vi "Msg Receive.vi"(11 "Self Actor in":refnum<class "Self Actor.lvclass">) -> (0 "error out":errorcluster, 1 "Destroyed Self?":bool, 3 "Self Actor out":refnum<class "Self Actor.lvclass">)   [LabVIEW 2021, in "LVCAM.lvlib" / "Self Actor.lvclass"]
uses:
  Self Actor.lvclass
  Msg Q/Msg Q.lvclass
  Msgs/LVCAM Nest Destroyed/LVCAM Nest Destroyed Msg/LVCAM Nest Destroyed Msg.lvclass
  Msg/Msg.lvclass
  C:/PPLs/LabVIEW-Composed-Actor-Model-LVCAM/LabVIEW-Composed-Actor-Model-LVCAM/AAM/Msgs/LVCAM Nest Destroyed/LVCAM Nest Destroyed Msg/LVCAM Nest Destroyed Msg.lvclass
  C:/PPLs/LabVIEW-Composed-Actor-Model-LVCAM/LabVIEW-Composed-Actor-Model-LVCAM/AAM/Msgs/LVCAM Nest Destroyed/LVCAM Nest Destroyed/LVCAM Nest Destroyed.lvclass
  C:/PPLs/LabVIEW-Composed-Actor-Model-LVCAM/LabVIEW-Composed-Actor-Model-LVCAM/AAM/LVCAM/Msg/Msg.lvclass
  C:/PPLs/LabVIEW-Composed-Actor-Model-LVCAM/LabVIEW-Composed-Actor-Model-LVCAM/AAM/LVCAM/LVCAM/LVCAM.lvclass
  C:/PPLs/LabVIEW-Composed-Actor-Model-LVCAM/LabVIEW-Composed-Actor-Model-LVCAM/AAM/Msgs/LVCAM Create Nest/LVCAM Create Nest/LVCAM Create Nest.lvclass
  C:/PPLs/LabVIEW-Composed-Actor-Model-LVCAM/LabVIEW-Composed-Actor-Model-LVCAM/AAM/Msgs/LVCAM Destroy Self/LVCAM Destroy Self/LVCAM Destroy Self.lvclass
  C:/PPLs/LabVIEW-Composed-Actor-Model-LVCAM/LabVIEW-Composed-Actor-Model-LVCAM/AAM/LVCAM/Msg Receive/Msg Receive.lvclass
  C:/PPLs/LabVIEW-Composed-Actor-Model-LVCAM/LabVIEW-Composed-Actor-Model-LVCAM/AAM/LVCAM/Msg Remain/Msg Remain.lvclass
  C:/PPLs/LabVIEW-Composed-Actor-Model-LVCAM/LabVIEW-Composed-Actor-Model-LVCAM/AAM/LVCAM/Propagate Error/Propagate Error.lvclass
  C:/PPLs/LabVIEW-Composed-Actor-Model-LVCAM/LabVIEW-Composed-Actor-Model-LVCAM/AAM/LVCAM/Self Actor Decorator/Self Actor Decorator.lvclass
  C:/PPLs/LabVIEW-Composed-Actor-Model-LVCAM/LabVIEW-Composed-Actor-Model-LVCAM/AAM/LVCAM/Read Self Actor/Read Self Actor.lvclass
  C:/PPLs/LabVIEW-Composed-Actor-Model-LVCAM/LabVIEW-Composed-Actor-Model-LVCAM/AAM/LVCAM/Self Actor/Self Actor.lvclass
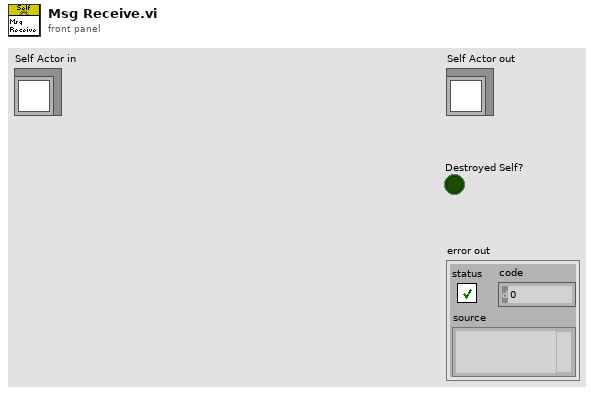
[diagram p1: front panel]
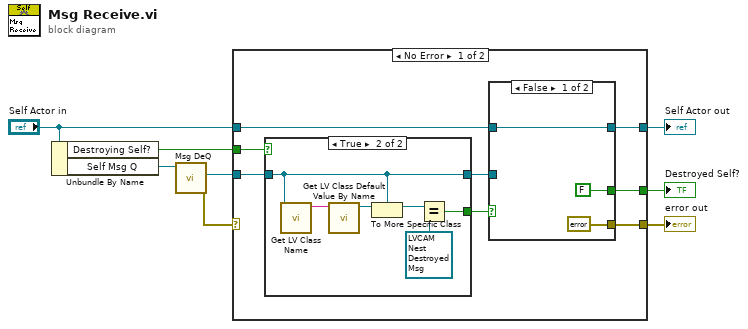
[diagram p0: block diagram]
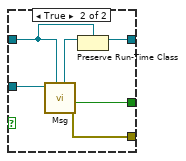
[diagram p2: hidden frame]
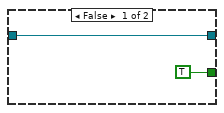
[diagram p3: hidden frame]
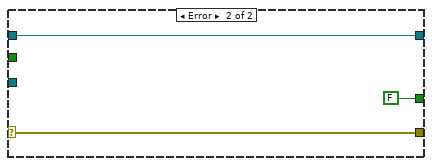
[diagram p4: hidden frame]
diagram:
  n1 = Unbundle By Name("Self Actor in") -> ("Destroying Self?"=w1:bool, "Self Msg Q"=w6:refnum<class "Msg Q.lvclass">)
  n2 = call "Msg DeQ.vi"("Msg Queue in"=w6) -> ("error out"=w7:errorcluster, "Msg"=w8:refnum<class "Msg.lvclass">)  [unwired: 9 in]
  n3 = case shown="No Error" w7 {
    selector: w7 -> [_ w35]
    tunnel: w8 -> [w10 _]
    tunnel: "Self Actor in" -> [w16 w36]
    tunnel: [w15 w35] -> w4
    tunnel: [w14 FALSE ("Destroyed Self?")] -> w3
    tunnel: [w13 w36] -> w2
    tunnel: w1 -> [w12 _]
    frame No Error {
      n4 = case shown="True" w12 {
        tunnel: [w27 w28] -> w11
        tunnel: w10 -> [w27 w28]
        tunnel: [TRUE w29] -> w9
        frame False {
        }
        frame True {
          n5 = call <vilib>:"Get LV Class Name.vi"("object"=w28) -> ("class name"=w33:string)  [unwired: 9 in, 1 out]
          n6 = call <vilib>:"Get LV Class Default Value By Name.vi"("class name"=w33) -> ("object"=w32:refnum<class>)  [unwired: 9 in, 1 out]
          n7 = To More Specific Class(target class=w28, reference=w32) -> (specific class reference=w30:refnum<class "Msg.lvclass">)  [unwired: 1 in, 1 out]
          n8 = Equal?(x=w30, y=refnum<class "LVCAM Nest Destroyed Msg.lvclass"> refnum ("LVCAM Nest Destroyed.lvlib:LVCAM Nest Destroyed Msg.lvclass")) -> (x = y?=w29:bool)
        }
      }
      n9 = case shown="False" w9 {
        tunnel: w16 -> [w17 w25]
        tunnel: [errorcluster {"status"=FALSE, "code"=0, "source"=""} ("error out") w24] -> w15
        tunnel: [FALSE ("Destroyed Self?") w23] -> w14
        tunnel: [w17 w22] -> w13
        tunnel: w11 -> [_ w20]
        frame False {
        }
        frame True {
          n10 = call-dynamic "Msg.vi"("LVCAM in"=w25, "Msg in"=w20) -> ("error out"=w24:errorcluster, "Destroyed Self?"=w23:bool, "LVCAM out"=w21:refnum<class "LVCAM.lvclass">)  [unwired: 7 in]
          n11 = Preserve Run-Time Class(object in=w21, 2:w25) -> (object out=w22:refnum<class "Self Actor.lvclass">)  [unwired: 1 in, 1 out]
        }
      }
    }
    frame Error {
    }
  }
  "error out" <- w4
  "Destroyed Self?" <- w3
  "Self Actor out" <- w2
